vi "Zero Power Meter.vi"(8 "error in":errorcluster, 11 "LTB-1 in":refnum<class "LTB-1.lvclass">) -> (0 "error out":errorcluster, 3 "LTB-1 out":refnum<class "LTB-1.lvclass">)   [LabVIEW 2018, in "LTB-1.lvlib" / "LTB-1.lvclass"]
doc: "This is a parent VI, the child VI will overwrite the functionality of this VI. \n\nThe purpose of the VI is to Tare/Zero the Power Meter. Programmatically, it must be confirmed that no input signal is injected into the system (or that the reference signal is input).\n\nAuthor: Ron Dexter\nCompany: Luminar\nModified: 5/20/2018"
uses:
  LTB-1.lvclass
  C:/AME Test Engineering/LabVIEW/PPLs/EXFO/Parent/EXFO.lvlibp/EXFO.lvclass
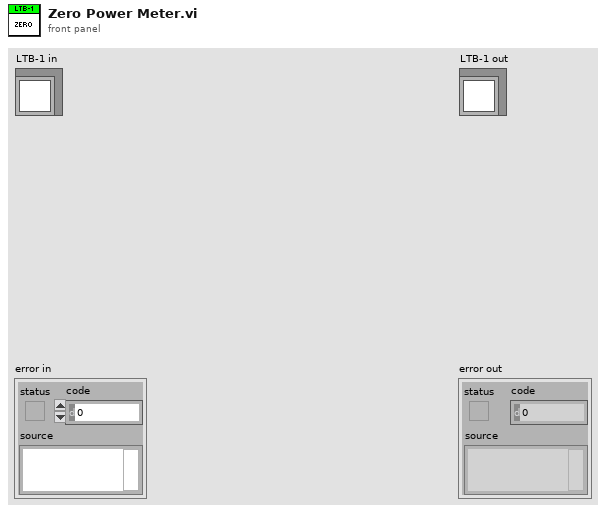
[diagram p1: front panel]
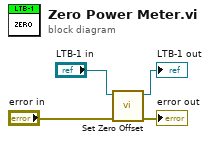
[diagram p0: block diagram]
diagram:
  n1 = call "Set Zero Offset.vi"("error in (no error)"="error in", "EXFO in"="LTB-1 in") -> ("error out"=→"error out":errorcluster, "EXFO out"=→"LTB-1 out":refnum<class "LTB-1.lvclass">)  [unwired: 8 in]
